vi "Parse.vi"(8 "Error In":errorcluster, 11 "object in":refnum<class "2021_10.lvclass">) -> (0 "Error Out":errorcluster, 3 "object out":refnum<class "2021_10.lvclass">)   [LabVIEW 2020, in "2021_10.lvclass"]
uses:
  2021_10.lvclass
  2021_10.lvclass/2021_10.ctl
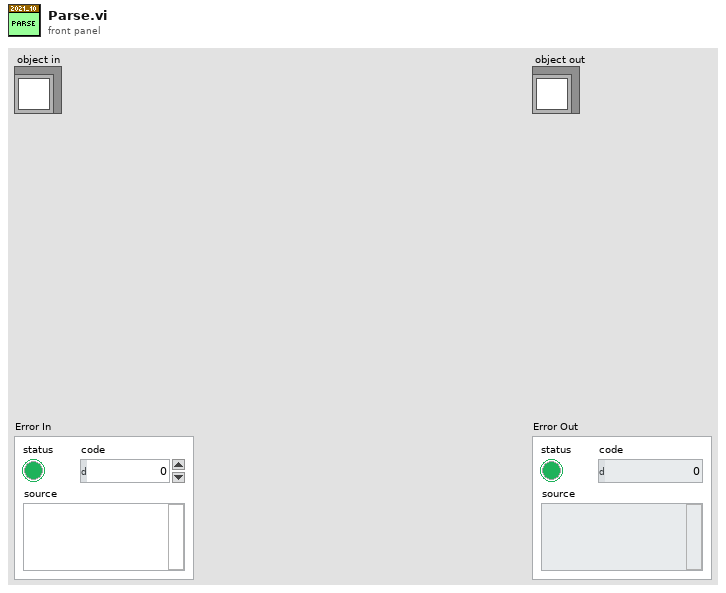
[diagram p1: front panel]
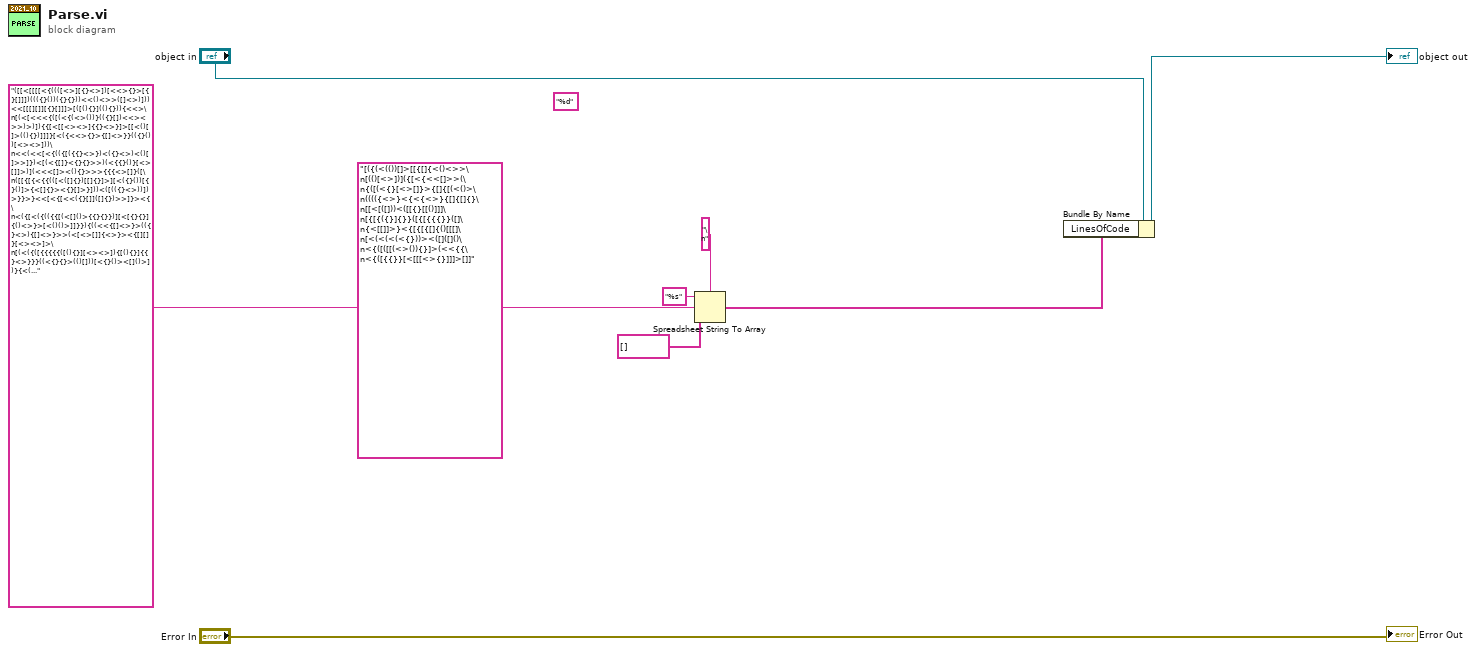
[diagram p0: block diagram]
diagram:
  (unwired) "[({(<(())[]>[[{[]{<()<>>\n[(()[<>])]({[<{<<[]>>(\n{([(<{}[<>[]}>{[]{[(<()>\n(((({<>}<{<{<>}{[]{[]{}\n[[<[([]))<([[{}[[()]]]\n[{[{({}]{}}([{[{{{}}([]\n{<[[]]>}<{[{[{[]{()[[[]\n[<(<(<(<{}))><([]([]()\n<{([([[(<>()){}]>(<<{{\n<{([{{}}[<[[[<>{}]]]>[]]" ("PuzzleInput")
  (unwired) "%d" ("format string")
  n1 = Spreadsheet String To Array(delimiter (Tab)="\n", format string="%s", spreadsheet string="([[<[[[[<{((([<>][{}<>])[<<>{}>[{}[]]])((({}())({}{}))<<()<>>([]<>)]))<<[[[][]][{}[]]]>[([(){}]((){})){<<>\n[(<[<<<{([(<{(<>())}(({}[])<<><>>)>)]){{[<[[<><>]{{}<>}]>[[<()[]>((){})]]]}[<({<<>{}>{[]<>}}(({}())[<><>]))\n<<(<<[<{(({[({{}<>})<({}<>)<()[]>>]})<[(<{[]}<{}{}>>)(<{{}()}[<>[]]>)](<<<[]><(){}>>>{{{<>[]}([\n([[{[{<{{(([<([]{})[[]{}]>][<({}())[{}()]>{<[]{}><{}[]>}]))<([(({}<>))])>}}>}<<[<{[<<({}[]]([]{})>>]}><{\n<({[<({(({{[(<[]()>{{}{}})][<[{}{}]{()<>}>[<()()>]]}}){((<<{[]<>}>(({}<>){[]<>}>>(<[<>[]]{<>}><{[][]}[<><>]>\n[(<({([{{{{{([(){}][<><>]){[(){}]{{}<>}}}((<{}{}>(()[]))[<{}()><[]()>])}{<({{}()}<<>{}])[{{}{}}{[]<>}\n({<<{{{{(((<({<>()})({{}}{{}{}})>{{([]{})<<>{}>}{<[]{}>{()[]}}}){[<[<>[]}[[][]]>{[{}[]]<<>()>}]<{({}<>)<{}\n[({{<<[{<({[<<{}{}>([][])><{(){}}>]{[[[]<>]][(<>()){{}}]}})(<[<{{}()}<<>[]>>([{}]{()<>})]>)>}[(<[({[<>[]]([]\n({[([(<([[<(({[]{}}{[]{}})<{()()}{<>()>>)[<{{}<>}>({[][]}(<>[]))]>]{(<{{[]{}}[[][]]}[[()[]][\n{([<{<{([<[[[[{}()]]]{<{[]()}((){})><[[]]<<>>>}][<<<{}<>>{()<>}>{<{}()>[{}[]]}>[(([]<>))[<[]{}>[[]]]]]>]<[\n<{[{{([[(<<<{({}{})(()<>)}[<{}()><{}<>>]>>>(<{{[{}()][(){}]}([[]()]([]<>))}{{<{}[]>{{}[]}}{[[]{}]{()\n{<{[<([{([[{{(<>[])[<>[]]}}][(<{[]()}<{}{}>>{<<>()>((){})])[{[<><>](()<>)}<<{}{}><<>[]>>]]])}])\n<[[[{<[<([[({[<>[]][()<>]}(({}[]){[]<>}))]])[([<<([])><<()[]>{<>[]}>><([()()]<[]()>){<<>[]><[]<>>}>]({<({}[]\n((<{{{[(({[[([()[]]([][]))(<[]<>>([]()))](((()())([]<>)){(()[])([]<>)})][{<([]{})<[][]>>{<[]{}>{(){}}\n(({{<[[{((((<<{}()>[()<>]>){[(()<>)([]())]})<{[<{}()>[[]()]]}<((<>())({}{}))[({}{}){{}<>}]>>))<[(({<\n[<{[{{({<[{[(<[]{}>{(){}})({{}<>}{{}{}})]<([[][]][[][]])((<><>)<<>()))>}<({{{}()}{{}{}}}(<[]{}>{()\n{{{{[{[{{<[[[{()<>}(<>[])]<{{}[]}[[][]]>]<<<<>>>>]{[[{()<>}<[]{}>]{{{}{})[{}[]]}]<(([]<>){{}()})>}>}[<([[({}\n([<<(({(<{{{<{()<>}>}}{(<({}<>){[]{}}>[<<><>><()()>])}}(<(({<>()}<(){}>){(<>{})[<>()]})>[(({<>[]}\n<{([[<{(((<(<[{}{}][(){}]>{<{}<>><[]<>>})<((<>())<()[]>)(<{}()>[[]<>])>>[(<[[]{}][[]()]>[<()()>[{}<>]]\n<[{{(<{[<(<[{[[][]]<()<>>)<(()<>)[<>()]>][<{{}{}}(<>[])>(<()[]>(()()))]>)<{<[{[]{}}]>[{<[]<>><<>{}>}]}[<{<\n[{((({({[<[<[(<>()){()[]}]([<>{}]{<>{}})>{[[[]<>][[][]]]{(()())[<>[]]}}]{{{{<>[]}{{}()}][([]\n<[{[<{(<((<{<{[]{}}(()<>)><(()<>){(){}}>}[{[{}[]]}<(()())[()()]>]>{{[<()[]>]{(<>[])<()()>}\n{<([<([{{{(({{()[]}}[([][]){(){}}]))}[[{{(<><>)<<>>}<<()()>>}][{[[[]<>]{(){}}]}<{{[]<>}<{}[]>}{{<>[]}<\n<<[<{{[<[<<([[{}<>]{[][]}][[{}{}](()<>)])[([{}]({}{}))[([]<>)<<>[]>]])<[<[()<>]>{[[]{}]<{}{\n[{[{<[({<((<[<<><>>(()<>)](<{}[]><<>()>)>[{([]())[()<>]}])([<([][])<()<>>>([<><>])]))[[{({<>[]}[()[]])}[[{(){\n{[([[<{[<{<{[(<>[])<{}()>](((){})([]<>))}[({<>[]}[()[]])([[]<>][{}{}])]><{{<()()>[()]}(<[]<>>[{}<>])\n{[<([(({([<[([()[]]<[]{}>){<{}<>>(()<>>}]([(()<>)([]())]((<><>)({}())))>]){[{(<[[]{}][(){}]>({[]{}\n[({<[{[<({<((<<><>>){[{}()]})<<{{}{}}[[]()]>(({}()))>>{[[{{}<>}({}<>)][(()<>)({}{})]]<{[()<>\n[([<{<{<{[(<[((){})[<>[]]]{{{}<>}[{}[]]}><[[()()][()()]]>)([[{[][]}{[]()}]]({<[]<>>(()<>)}[[[]<>]({}<>)]))\n<([<{[<<[<(<{{(){}}({}{})}[<<>()>(<>())]>[<<[][]>([]())>{[<><>]<{}()>}])>]{{[{[<{}{}>(<>{})][[<>()]<<>[]\n<{([<<(<{{[{<[(){}]{[]}>((<>[]){()[]})}(<{<>}(()())>(<<>[]><<><>>))]<[<<[][]>([])>]>}}{[<<(<[]>{<>[]])(<()<>>\n(<{([<{[(<<(<[(){}]({}())><{()[]}<[]()>>){[<<><>>[{}[]]]<({}<>)[[]<>]>}>{[[([]{})<{}[]>]][{<[]\n<<({[<({<{[((({}))<(<>[])>)<[[<><>]([]())]>]}<{[<{(){}}(()())><<[]<>>{()[]}>]}>>[<{{{<()()>[[]()]}(<\n[{[{<{[[{{{[<[(){}]{<><>}>(({}[]))]}<(<[[]<>]{<><>}>{(()){(){}}}>[({()()}<{}[]>)]>}}]{<((<{<(){}><{}<>>}\n{([((<<([{<[[([][])<{}[]>][[(){}]{[]<>}]](<{[]{}}<<><>>>)>[{{{<>{}}([]{})}[<[]()>(()())]}{<(<\n<{{((<{{({{<(<(){}>({}<>))[[{}[]]{[]{}}]>{[{(){}}{()[]}]({<>[]}<[][]>)}}([(<(){}>[[]<>])[[{}{}]<{}<>>]\n[<[<({[<{{{{{<<>[]>}({<>()})}}([[(()<>)<()()>]]>}([(((<>{}))[[<>[]][()[]]])<{([]{})(()[])}>]<{\n<<[<{<{({<([({{}[]}){{{}()}{{}{}}}]<[{()()}<<><>>]{(<>())(()())}>)(<{({}<>)([]{})}(<<>{}><[]()>)>{\n([{({{<<<{{{((()[])(<>[])){(()[])[()<>]}}(((<>{})<()()>))}<<[{<>{}}{{}[]}]<(<><>){<>[]}>>(<{<>[]}<(){}>>)>\n{[[(<({{[<<([<()[]>[(){}])<<[][]>[<><>]>)({({}())([]{})}[{{}()}({})])><<{{[][]}[()[]]}{{{}()}{<>[]}}\n<(<[{<<{[{<({{()<>}[{}[]]}[<{}>({}<>)])<[{(){}}(<><>))>>[<{<[]{}>[{}()]}<[()]<<><>>>><{<{}{}>[[]<>]}[<()[]>(\n<([{{{([<(<(<[()()]{[]()}>{[()()]{{}{}}}){[[[]<>]{[]{}}]<<()<>>>}>)[[{(({}<>)<<><>>)[[()()]{[]()}]}(<[(){}]{<\n{[<{{<(<{<<[<(<>())({}())>[[()]{[]()}]]({{[]()}}<<[][]>{<>{}}>)>>(([[[{}[]]((){})]([[]{}]{\n<<<<(<{{<((<[<()()>{<>[]}]>)[[<({}())<(){}>>]{(<(){}><<>()>)[{<>[]}[{}<>]]}])(([<<<>{}>>[{[][]}{{}{}}]]{<[\n([[<<<({[[(<([<><>]{<>()})>(([<>][{}<>])<[[][]>([]{})>))({{<[]>{<>()}}{<[][]>[[]{}]}}<[{[]{}}{{}{}}\n{[[<<(<<([(([{<>()}<<>()>]{[{}[]]{()[]}}){[[(){}){(){}}]{<<>[]>{[]<>}}})[<([[]]<<>{}>)>{{{<>{}}<<><>>}[[\n(<{{<([[[([[(<()()>[[]<>]){[{}]{[][]}>]])[<[{(<>)(()[])}({<>[]}[{}()])]{<[<>{}]{{}()}>{{()}{<>{}}}}>([\n{<[{(((([<[{{<<>()>[()()]}<([]())<[]()>>}<((<>))[<[]{}>{[]<>}]>){{([()]<<>[]>)[<[][]>{()}]}[{((){})\n((<{<{<(((<(({(){}}([][])){((){})<[]>})({(()[])(()())}{{()<>}[<>{}]})>[(<[()]<[]{}>>(([][]){<><>\n{{{({[{(<<<<[[(){}]<<><>>]([[]{}]<{}[]>)>>>>[{{<[{<><>})[(<>[])[{}{}]]>{{<<><>>}({<><>}{()()})\n{{[{[(({[(({<[{}{}]>[{[]<>}[{}()]]}(((()<>)<()[]>))){{{<{}[]>{{}<>}}{{{}<>}}}<<<{}{}>>(({}()))>})({<<{\n{<{<[<(<{<[(<({}{})[[]{}]>{([]<>)[<>[]]})>([<{<>()}{[][]}><{()[]}<[][]>>][<{{}{}}{[]()}>[<<><>>[{}<>]]]\n{({{[<(<[[<[[({}{}){<><>}]](({()<>}{{}<>}){({}<>)<()[]>})>]}><<<{{(({}{})<()()>)([{}[]][<>[]])}\n(<<{<<{{[{((({[]{}}))<([<>()]{{}{}})(<{}{}><[]<>>)>)[{({{}{}}<()>)}([<{}[]>([]())]{<<>[]}([]{})})]}<\n{{<{([[<[(<[[<{}<>>]({[][]}<<>{}>)][[[()<>][<>[]]]{[[][]]}]>(({([])[<><>]}[(()<>)<(){}>])<<[{}]{<\n<{{{[<{[<<[<{[<><>]{[]{}}}[<{}()>{{}[]}]><<<[][]>{{}()}><(<>())[<>[]]>>]<[[<()[]>[<>[]]](({}<>))]>>]]}>]{([<(\n[<{({{[{<<{<<[()<>]<<>()>>([<>[]]([]()))><[<<>{}>{{}{}}]>}(<{[()()][()()]}(([]{}))>)>([(({{}()}<[]{}\n(<{{({({({<<((()<>)(()()))[(<>[]){<>[]}]>({({}[])[<>{}]})>})}){[[({{(<()<>>{<><>})<{<>[]}<{\n[[<<<{<<[<[[{<{}{}>(<>{})}]{([[][]][[]{}])<([]<>)<[]{}>>]]>[[<[[()[]]({}())](([]())[()<>])>\n{[(<[[{({<{<[{(){}}]{[[][]]<()[]>}>}}[([<[{}[]]([][])><<[]()>[()()]>]({<()<>>(<>[])}<<(){}><<><>>>)\n[{(<<{{[<{{{[[(){}]({}())]<(<>[])>}<{{()<>}(<><>)}>}}[(((([]())[(){}])(({}<>)<()()>))[<(<><>)<[]{}>>\n<<<{<([[[({{<([]{})[{}()]>[([]<>)[[]()]]}(<<<><>>>)}[[{<()[]>({}<>)>]([[<><>]][(())[[]()]]\n([{{([<<<{{(<[{}[]][{}()]><[<>()]{[]()}>)({{[]<>}[{}()]>({()<>}<{}()>))}[<<<{}<>>{[]()}>>]}>>>\n{[<{{<{{<[[<({()[]}{<>{}}){{<>[]}{(){}}}>]]<([[[[]{}]{{}{}}][<{}()><[]{})]])({((<><>)[()[]])<[[]]<{}<>>>}[\n[[{(<<{<{<{<((<><>)[<><>])>}>({<(<[]()>[(){}>)>{{[[][]]}{{()()}{()()}}}})}{[{{((()())((){}))(({}\n[{[<{[((<<[(<<<>[]>({}[])>(<<>>{<>[]})){{({}())[{}<>]}{{<><>}{<><>}}}][[{({}<>)}({<>()}[(){}])]\n<<([[{([{{<<<<{}()>({}())>([()()])>(<([][])><<()[]>>)>}}{<{[<[<>{}][<><>]>]<[(()())[()<>]]<{{}{}}{[]<\n{{[<{{[{{{<{<<<>[]><()<>>>(<{}<>><{}{}>)}<[((){})[[]{}]]{<{}>}>>}<[[([{}[]]{[]<>})][([()<>]<{}\n[(([(((<{[{{<[[][]](<>{})><{{}[]}[(){}]>}{(({}[])([][]))<[{}[]][[]]>}}([[{[]}(()[])][([]<>){()\n{[<{<<[<{([<({[]<>}[()]){[[]()]([]())}>{([<>]{<>{}})}])<(([({}[]){[]<>}]{([]<>)[[]<>]}){{<(){}}[{}[]]}([[]{\n[{<<<[<[{(<{({{}{}}[[]()])([[]()])}>)[[(({<>}({}())){{<>[]}<[]<>>})[(<<>{}>)]]]}{<[[[[{}()}(<>())]{<<><>\n((([{[<({([[((<><>)[{}()])(({}<>)({}()))]{[<<>{}><<>()>]({()()}[<>])}]<[{[{}()]}([{}{}]<()()>)]>)}<([<[{[]\n(<[<{[<[{[[<[<{}()>[[]]]>{{<<>>({}[])}<{{}<>}>}][({<()()>[()[]]>({[]()}))]]}]({<({<[{}()]{{}()}>{[()<\n(<<([{<[<(<[[{[][]}[(){}]]]}<{{<{}{}>}{(()[])(()())}}>)>][[{[([([][])(<>())](<()>[[]()]))(<{[]()}{()\n[{{<<<<{(({{({{}[]}<()[]>)({{}()}{<>()})}<[(<>())]{(<><>)}>}((([<>()]{{}[]})[<<>[]>(()[])])[(<{\n<[[{<([[<[{(({<>[]}({}()))(<[]<>>{<><>}))<[(<>[])(()<>)]{{(){}}{{}<>}}>}([[{()()}(()())]]((<[][]>([]()))(<\n(<(<[{<([[({<<(){}>[{}()]>[<[]>[()()]]}(<<{}{}><[]<>>>({{}[]})))<[({[]()}[{}<>])<(()<>){[][]}>]{([\n{(<(((<[<<<[[(()())[{}]]({<>()}({}()))]<<{()()}(()())>[{<>[]}[[]<>]]>>>([{(<{}{}>{{}})<[{}[]](<><>)>)[<[<>\n<[<([<{<<<{{{<()[]>{<>[]}}[<[][]>[{}()]]}}<{{{[]<>}<[]{}>}<{{}()}[()()]>}>>)>[([<{((<>{})[()(\n<<[<<{([[[[<[([][])((){})][{{}()}({})]>([{{}{}}(<>[])])]{{(<<>[]>{()[]}){[<>()]{[][]}}}[{{<>}<{}<>>}<<{}()>((\n{{(<{[<<[{[(<<[]>(<><>)>[{[]()}{<>{}}))<{({}[])<[]{}>}{(<>{})[[][]]}>]<(([<>{}]([][]))<[[][]][<>\n(({([{({<[<<{([]())(<>())}([<>{}])><({<>})<<<><>>>>>[<{[{}<>]{[][]}}<{()()}<[]{}>>>[{<()<>>{{}}}\n<{[{({[(({[((<()>{()<>}))<([()[]]<<>()>)[{(){}}([])]>](({<()[]><{}<>>}({{}}([][]))))}))<<[[[[{(\n[{<([[({{{{({([][])[<>{}]})[{({}{}){<>{}}}]}({[{[]{}}([])]({()()}<[]{}>)}<[[{}{}][{}[]]]{<(){}>{<><\n(<[{{{{[{(((<[[]())([]())>{<()()><[][]>})){<(<<>{}>[[]()]){{<>{}}[<><>]}>[<{<>()}<{}{}>>{<()[]\n({{[{[[[{<{([<{}<>>[{}()]])(({()[]}{()[]}){<{}<>>{()}})}<<{[<><>]}<[()[]>{{}<>}>><((()[]))>>>\n{<[(<{[(([({<[<>[]]<<><>>}[[<>()]{{}<>}]}[{<{}>}<[()<>]<[]()>>])(<[[<>()]{{}()}]<({}[])[{}()]>>([[<>{}]<<\n{<[<{{(([{[[{<[][]>[<>[]]}<[{}<>]<<>{}>>]]{<(([]<>))((<>{})[<>{}])>{(<{}<>>[<>])([(){}]{<><>})}}}[{[({{}<>\n<<({[(<{<[{{[<{}[]>]<[<>{}]{[]<>}>}}<([{[]<>}]{(<>{})}){(<[]<>><()>)[<()()>([]{})]}>](([{{[][]}[{}[]]}[{<>[\n[<[[[[<({([[[[<>()]{{}()}][{<>{}}{[]}]]<{<{}>{<>)}>]{[<[<><>]{()()}><((){})(()())>]{(({}[])){[()()](\n{<[[[<<<<<{[<[<><>]<()<>>>{{()[]}[{}()]}]<<[<><>]{()()}>>}({{{<>()}([]<>)}[[(){}][()[]]]})>>>>>]\n(<[{{[[{({[{<{<>[]}[<>[]]>}]})}{{({{{([][])((){})}(({}[]))}([{<><>}(()[])]({<>{}}<{}>))}{([((\n<[[(<{({<<{{[{<><>}]<(<>{})<<>()>>}[<([]<>)(<>[])>[<{}<>><[]<>>]]}<({{{}<>}[()<>]}{[<>[]][[]\n{{<[[<<<{{{(<[{}()]>[<(){}}(()[])])[[{(){}}<{}()>][({}[])([]{})]]}}[<<<[()()]{[][]}><<[]>>>{<<{}[]>{<>[]}>[<\n((<<{([[([[<([[]{}]<[]{}>)>]](<({{{}{}}([][])}{(<>())[<><>]})[((()())[{}{}])[(<>{})[[]<>]]]>))[{{({{{}{}}[<\n<<<(<(<[[<(<[{()[]}<{}{}>]>([{[]()}[()[]]]<(<>())>))[{({<>{}><{}<>>)}{[[{}()](())]<<()[]><<><>>>}]>{{<(\n{{{<(({{[(({{<[]()><<>>}{[()[]]{<>{}}}})({<<()]<[]{}>>}([[()()]{[]<>}]))){<(<(<>()){[]<>}>[\n[({([{<(<[<{[<<>[]>[[]]]{[{}[]]<(){}>}}{<<[]()>({}())>([[]{}][[]()])]>]<<{{[{}{}][[]{}]}{{(){}\n<{{<[[([[(<{{{<>[]}[()<>]}(<[]{}>)}<{[{}{}]({}{})}>><{[{{}[]}(<>{})]<{<><>}<{}{}>>}>)][<{({[(){})<()()>})\n<<{{[{{[[{{[({{}[]}[()[]])({[]<>}{{}()})](<<<>[]>{[]<>}>{{()[]}[<>()]})}}](<{{{<<><>><{}[]>}}}({\n[<[<<(<[((((<(<>[]}<[]>><{[][]}({}{})>))[<{[[][]]}([{}<>][{}])>[<{[]()}({}{})>{(()()){{}{}\n[<<{[([[([{<[{(){}}[{}{}]]><{[[]<>][(){}]}<{[]{}}[()()]>>}({((<>))<{()}<[]{}>>}{[[[]]{<><>}]<[[]<>]\n[[[{<([{[<[<{[<>()]<()<>>}<{<>()}<[]<>>>>([(<>{})(<>[])]<<(){}><[]<>>>)]({{[<>{}]}({<>[]}<()[]>)}[(<{}<\n{<<[[{([{((({[{}()]{()[]}}[<{}>[{}{}]]))({[<(){}><()[]>]}))}])[<(<([([<>{}))<[[][]]{(){}}>])(\n[{(<<{<[[{<[{[{}[]](()<>)}[[{}{}][[]<>]]]><(<(<>[])({}())>[{{}{}}<<>()>>)>}<{(<<{}[]>[[]()]>{<\n<{(((([<{[{[<<(){}>[()<>]>{<{}>({}())}]{[{<>()]({}{})]}}][(<<{()()}>({[][]}<{}[]>)>)]}[(<[{(\n([<((<<[([[[<[()()]<{}()>>]<(<()()>[[]])[<{}<>>((){})]>}{({((){}){[]{}}}[[[]]<{}<>>])(<{()[]}[()[\n{((<[({<<({(<{<>[]}{[][]}>){<<()()>{[][]}><{[]{}}>}}<<[<[]>(<>())]<<<>{}>{{}()}>>[[[<>{}]<()()}]<\n[[<{{{({([((<[()<>]<{}>><(()[])[{}()]>)[({<><>}({}))<<{}<>><[]{}>>]){[([{}<>](()()))]<[{()\n{<<[[{[[[[[[[[<>()][{}]]<(<>())(()[])>]]<{[<[]<>>({}{})]}<[({}())][{{}()}{{}[]}]>>]<[[(<()()>{[]{}})" ("PuzzleInput"), array type (2D Dbl)=string[] []) -> (array=w2:string[])
  n2 = Bundle By Name(cluster="object in", "LinesOfCode"=w2) -> (→"object out":refnum<class "2021_10.lvclass">)
  "Error Out" <- "Error In"
